vi "qWOS.vi"(0 "System no.":i32=1 min=1 max=4 step=1, 2 "Generator ID":i32[](array[numeric]) min=1 step=1, 3 "All generators?":bool, 5 "error in":errorcluster) -> (14 "Offset":dbl[](array[numeric]) format="%.6f", 19 "error out":errorcluster)   [LabVIEW 2026]
doc: "Returns wave generator output offset.\n\nC-413: Generator ID can be 1 to 2.\n\nE-517, E-518: Generator ID can be 1 to 3.\n\nE-709: Generator ID can be 1\n\nE-712: Generator ID can be 1 to No. of connected axes\n\nE-725, E-727: Generator ID can be 1 to No. of connected axes\n\nE-753: Generator ID can be 1\n\nE-754: Generator ID can be 1"
panel:
  # "Returns wave generator output offset."
  # "Query"
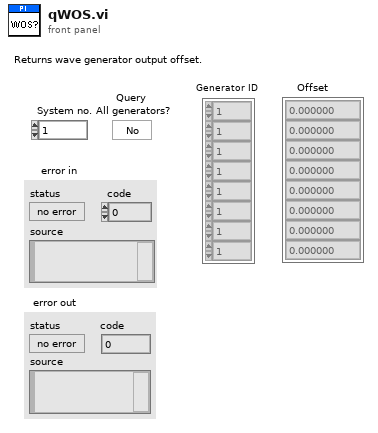
[diagram p1: front panel]
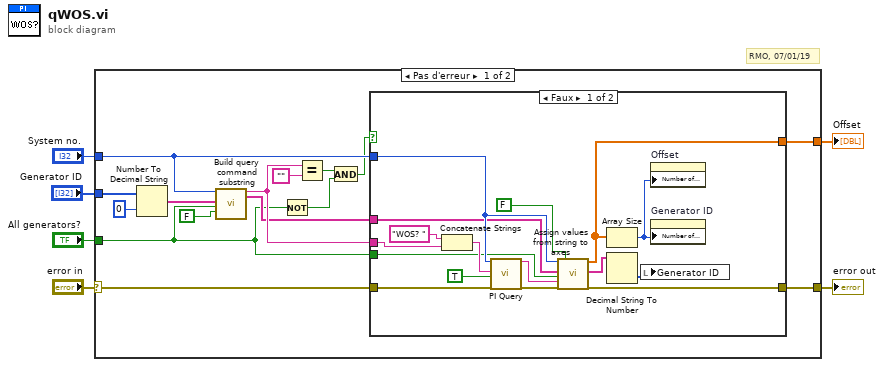
[diagram p0: block diagram]
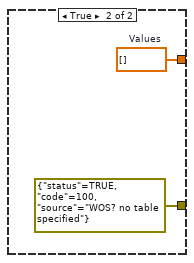
[diagram p2: hidden frame]
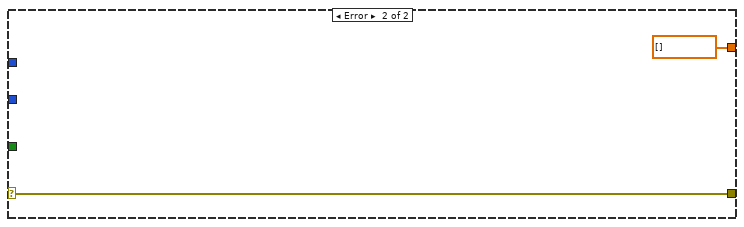
[diagram p3: hidden frame]
diagram:
  # "RMO, 07/01/19"
  n1 = case shown="Pas d'erreur" "error in" {
    selector: "error in" -> [w9 w40]
    tunnel: [w15 dbl[] [] ("Values")] -> w6
    tunnel: "Generator ID" -> [w11 _]
    tunnel: [w8 w40] -> w4
    tunnel: "System no." -> [w19 _]
    tunnel: "All generators?" -> [w13 _]
    frame No Error {
      n2 = Number To Decimal String(number=w11, width (-)=i16 0) -> (decimal integer string=w10:string[])
      n3 = call "Build query command substring.vi"("System no."=w19, "Axes to query in"=w10, "Query\nAll axes?"=w13, "For all axes: use\nAxis identifier?"=FALSE ("For all axes: use\nAxis identifier?")) -> ("Command substring"=w20:string, "Axes to query out"=w18:string[])  [unwired: 2 in, 12 out]
      n4 = Not(x=w13) -> (.not. x?=w17:bool)
      n5 = Equal?(x=w20, y="" ("x")) -> (x = y?=w16:bool)
      n6 = And(x=w16, y=w17) -> (x .and. y?=w7:bool)
      n7 = case shown="Faux" w7 {
        tunnel: w20 -> [w34 _]
        tunnel: w19 -> [w33 _]
        tunnel: w18 -> [w32 _]
        tunnel: [w31 w38] -> w15
        tunnel: w13 -> [w29 _]
        tunnel: w9 -> [w25 _]
        tunnel: [w24 errorcluster {"status"=TRUE, "code"=100, "source"="WOS? no table specified"} ("error out")] -> w8
        frame False {
          n8 = Concatenate Strings("WOS? ", w34) -> (w35:string)
          n9 = call "PI Query.vi"("System no."=w33, "String to send"=w35, "Attach termination char.?"=TRUE ("Attach Linefeed?"), "error in"=w25) -> ("String read"=w22:string, "error out"=w23:errorcluster)  [unwired: 3 in, 11 out]
          n10 = call "Assign values from string to axes.vi"("System no."=w33, "Queried axes"=w32, "All axes queried?"=w29, "Input String"=w22, "error in"=w23, "Axes related?"=FALSE) -> ("Values"=w31:dbl[], "Queried axes out"=w27:string[], "error out"=w24:errorcluster)  [unwired: 3 in, 8 out]
          n11 = Array Size(array=w31) -> (size(s)=w28:i32)
          n12 = Decimal String To Number(string=w27) -> (number=w26:i32[])  [unwired: 3 out]
          n13 = local write "Generator ID"(w26) -> ()
          n14 = property on="Offset" class="Tabl (strict)"("Number of Rows"=w28) -> ()  [unwired: 2 in, 2 out]
          n15 = property on="Generator ID" class="Tabl (strict)"("Number of Rows"=w28) -> ()  [unwired: 2 in, 2 out]
        }
        frame True {
          w38 = dbl[] []  # Values
        }
      }
    }
    frame Error {
    }
  }
  "error out" <- w4
  "Offset" <- w6
